vi "_unittest Assert Tolerance.vi"(4 "Ignore Error? (F)":bool, 6 "Assert Error Code (0=No error)":i32, 7 "Message":string, 8 "error in (no error)":errorcluster, 10 "Tollerance (1E-5)":dbl=1e-05, 11 "Actual Value":dbl) -> (0 "error out":errorcluster)   [LabVIEW 2019, in "labview_json_tests.lvlib"]
uses:
  labview_json_tests.lvlib
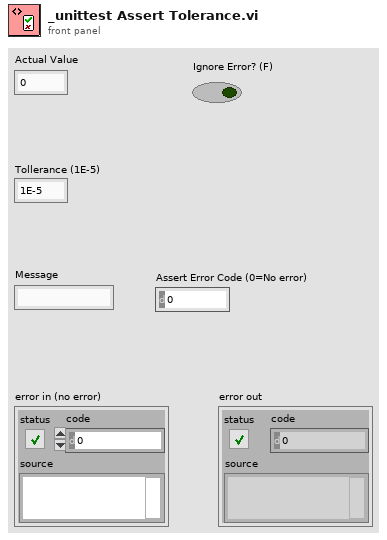
[diagram p1: front panel]
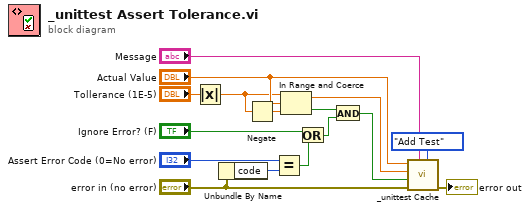
[diagram p0: block diagram]
diagram:
  n1 = Absolute Value(x="Tollerance (1E-5)") -> (abs(x)=w3:dbl)
  n2 = Unbundle By Name("error in (no error)") -> ("code"=w16:i32)
  n3 = Negate(x=w3) -> (-x=w2:dbl)
  n4 = Equal?(x="Assert Error Code (0=No error)", y=w16) -> (x = y?=w7:bool)
  n5 = In Range and Coerce(upper limit=w3, x="Actual Value", lower limit=w2) -> (coerced(x)=w5:dbl, In Range?=w1:bool)
  n6 = Or(x="Ignore Error? (F)", y=w7) -> (x .or. y?=w13:bool)
  n7 = And(x=w1, y=w13) -> (x .and. y?=w10:bool)
  n8 = call "_unittest Cache.vi"("Action"=enum8{"Report", "Add Test Case", "Add Test"}."Add Test", "Message"="Message", "error in (no error)"="error in (no error)", "Passed?"=w10, "Second Value"=w5, "First Value"="Actual Value") -> ("error out"=→"error out":errorcluster)  [unwired: 4 in, 1 out]
